vi "Write Controller Data.vi"(10 "Controller Data":T1 {"Force Error" min=-888.0 max=888.0 format="%.2f"; "Force Demand" min=-888.0 max=888.0 format="%.2f"}, 11 "Logger in":refnum<class "TestDataLog.lvclass">) -> (3 "Logger out":refnum<class "TestDataLog.lvclass">)   [LabVIEW 2015]
uses:
  TestDataLog.lvclass
  Typedefs/ForceDemand.ctl
  Typedefs/M1M3SSSTypedefs.lvlib
  Typedefs/ControllerData.ctl
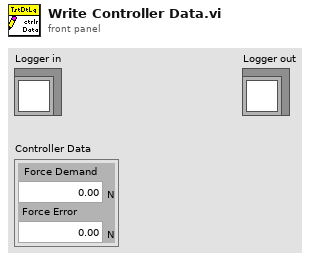
[diagram p1: front panel]
types:
  T1 = typedef "M1M3SSSTypedefs.lvlib/ControllerData.ctl" = cluster{"Force Demand":T2, "Force Error":T2}
  T2 = typedef "M1M3SSSTypedefs.lvlib/ForceDemand.ctl" = dbl[unit]
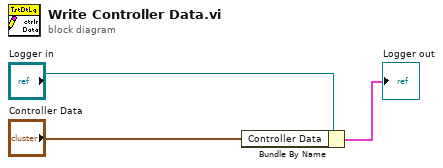
[diagram p0: block diagram]
diagram:
  n1 = Bundle By Name(cluster="Logger in", "Controller Data"="Controller Data") -> (→"Logger out":cluster{})
